vi "HeaderInfo.vi"(0 "refnum":refnum<file>, 11 "offset":i32) -> (2 "header info":cluster{"Header":string, "Head length":i16}, 4 "dup refnum":refnum<file>, 6 "Header Version":string, 8 "header length":i16, 10 "blank":i16)   [LabVIEW 2022 SP3]
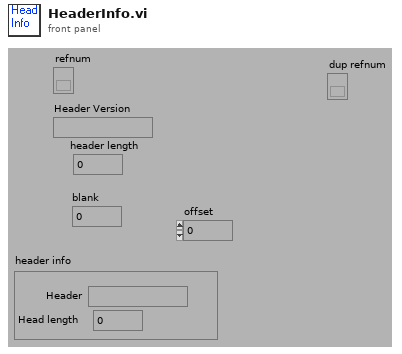
[diagram p1: front panel]
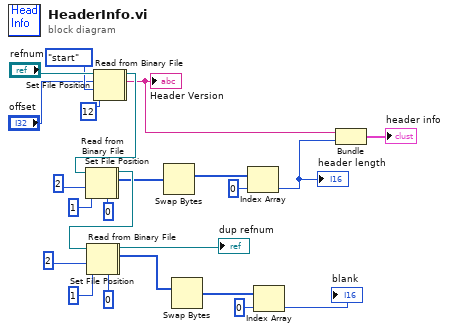
[diagram p0: block diagram]
diagram:
  n1 = Set File Position(offset (in bytes) (0)="offset", refnum="refnum", from (0:start)=enum16{"start", "end", "current"}."start" ("pos mode (0:2)")) -> (refnum out=w2:refnum<file>, error out=w1:errorcluster)  [unwired: 1 in]
  n2 = Read from Binary File(8:w1, 10:12 ("count"), 11:w2) -> (2:w15:string, 3:w26:refnum<file>)  [unwired: 5 out]
  "Header Version" <- w15
  n3 = Set File Position(refnum=w26, from (0:start)=2) -> (refnum out=w4:refnum<file>, error out=w3:errorcluster)  [unwired: 1 in, 1 out]
  n4 = Read from Binary File(5:i16 0 ("byte stream type"), 8:w3, 10:1 ("count"), 11:w4) -> (2:w17:i16[], 3:w25:refnum<file>)  [unwired: 4 out]
  n5 = Set File Position(refnum=w25, from (0:start)=2) -> (refnum out=w6:refnum<file>, error out=w5:errorcluster)  [unwired: 1 in, 1 out]
  n6 = Read from Binary File(5:i16 0 ("byte stream type"), 8:w5, 10:1 ("count"), 11:w6) -> (2:w16:i16[], 3:→"dup refnum":refnum<file>)  [unwired: 4 out]
  n7 = Swap Bytes(anything=w17) -> (byte swapped=w14:i16[])
  n8 = Swap Bytes(anything=w16) -> (byte swapped=w12:i16[])
  n9 = Index Array(array=w14, index=0 ("Index")) -> (element=w9:i16)
  "header length" <- w9
  n10 = Index Array(array=w12, index=0 ("Index")) -> (element=→"blank":i16)
  n11 = Bundle(w15, "byte stream type"=w9) -> (→"header info":cluster{string, "byte stream type":i16})  [unwired: 1 out]
